vi "RecordOpen.vi"(0 "PATH":string) -> (1 "refnum out":refnum<file>, 2 "current time":u32)   [LabVIEW 2014]
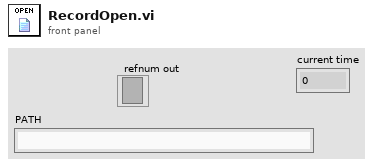
[diagram p1: front panel]
types:
  T1 = enum16{"open", "replace", "create", "open or create", "replace or create", "replace or create with confirmation"}
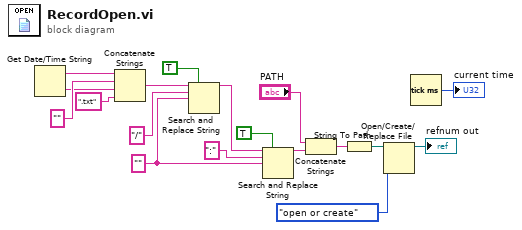
[diagram p0: block diagram]
diagram:
  w8 = "" ("replace string (\"\")")
  n1 = Get Date/Time String() -> (date string=w14:string, time string=w17:string)  [unwired: 3 in]
  n2 = Concatenate Strings(w14, "" ("string"), w17, ".txt" ("string")) -> (w7:string)
  n3 = Search and Replace String(replace all?=TRUE ("replace all? (F)"), input string=w7, search string="/", replace string=w8) -> (result string=w11:string)  [unwired: 4 in, 3 out]
  n4 = Search and Replace String(replace all?=TRUE ("replace all? (F)"), input string=w11, search string=":" ("replace string (\"\")"), replace string=w8) -> (result string=w6:string)  [unwired: 4 in, 3 out]
  n5 = Concatenate Strings("PATH", w6) -> (w5:string)
  n6 = String To Path(string=w5) -> (path=w16:path)
  n7 = Open/Create/Replace File(file path (use dialog)=w16, operation (0:open)=T1."open or create") -> (refnum out=→"refnum out":refnum<file>)  [unwired: 4 in, 2 out]
  n8 = Tick Count (ms)() -> (millisecond timer value=→"current time":u32)
